vi "Uint32Array Create.vi"(8 "error in (no error)":errorcluster, 11 "U32 array in":u32[](array[numeric])) -> (0 "error out":errorcluster, 3 "Uint32Array DVR out":refnum<data-value>)   [LabVIEW 2015, in "MDSplus.lvlib"]
uses:
  <vilib>/MDSplus/Library/MDSplus.lvlib
  <vilib>/MDSplus/Classes/Data_Class/Array_Class/Uint32Array_Class/Uint32Array.lvclass
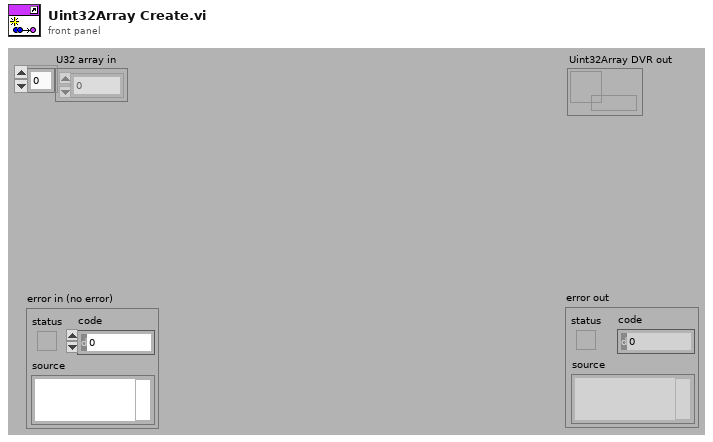
[diagram p1: front panel]
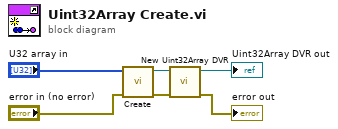
[diagram p0: block diagram]
diagram:
  n1 = call <vilib>:"Create.vi"("error in (no error)"="error in (no error)", "U32 array in"="U32 array in") -> ("error out"=w3:errorcluster, "Uint32Array out"=w4:refnum<class "Uint32Array.lvclass">)  [unwired: 8 in]
  n2 = call <vilib>:"New Uint32Array DVR.vi"("error in (no error)"=w3, "Uint32Array in"=w4) -> ("error out"=→"error out":errorcluster, "Uint32Array DVR out"=→"Uint32Array DVR out":refnum<data-value>)  [unwired: 8 in]
